vi "NonLinearPidTuningPanel.vi"() -> (3 "Output":string)   [LabVIEW 2014]
uses:
  <vilib>/silver_ctls/ArrayMatrixCluster/Real Matrix NI_Silver.ctl
panel:
  in  "Matrix Type":u16(ring) items=["Diagonal", "Normal"]
  in  "K anti wind up":T1=[[2.0, 0.0, 0.0, 0.0, 0.0, 0.0], [0.0, 1.0, 0.0, 0.0, 0.0, 0.0], [0.0, 0.0, 2.0, 0.0, 0.0, 0.0], [0.0, 0.0, 0.0, 0.0, 0.0, 0.0], [0.0, 0.0, 0.0, 0.0, 0.0, 0.0], [0.0, 0.0, 0.0, 0.0, 0.0, 1.0]]
  in  "Ki":T1=[[10.0, 0.0, 0.0, 0.0, 0.0, 0.0], [0.0, 10.0, 0.0, 0.0, 0.0, 0.0], [0.0, 0.0, 20.0, 0.0, 0.0, 0.0], [0.0, 0.0, 0.0, 0.0, 0.0, 0.0], [0.0, 0.0, 0.0, 0.0, 0.0, 0.0], [0.0, 0.0, 0.0, 0.0, 0.0, 5.0]]
  in  "Kd":T1=[[400.0, 0.0, 0.0, 0.0, 0.0, 0.0], [0.0, 400.0, 0.0, 0.0, 0.0, 0.0], [0.0, 0.0, 400.0, 0.0, 0.0, 0.0], [0.0, 0.0, 0.0, 0.0, 0.0, 0.0], [0.0, 0.0, 0.0, 0.0, 0.0, 0.0], [0.0, 0.0, 0.0, 0.0, 0.0, 200.0]]
  in  "Kp":T1=[[300.0, 0.0, 0.0, 0.0, 0.0, 0.0], [0.0, 300.0, 0.0, 0.0, 0.0, 0.0], [0.0, 0.0, 500.0, 0.0, 0.0, 0.0], [0.0, 0.0, 0.0, 0.0, 0.0, 0.0], [0.0, 0.0, 0.0, 0.0, 0.0, 0.0], [0.0, 0.0, 0.0, 0.0, 0.0, 200.0]]
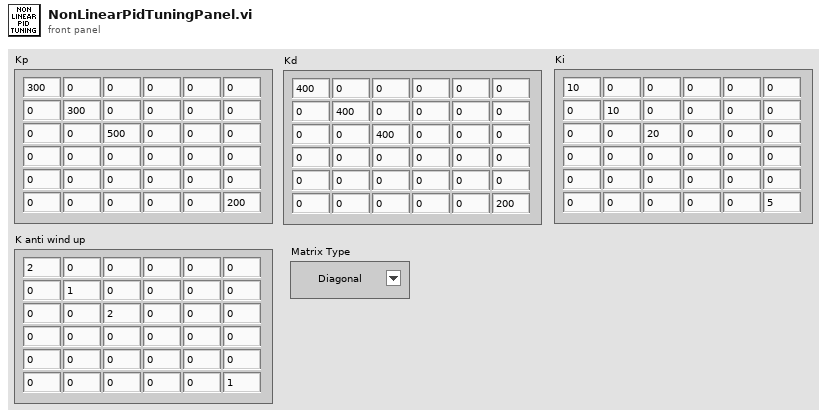
[diagram p1: front panel]
types:
  T1 = typedef "Real Matrix NI_Silver.ctl" = dbl[][]
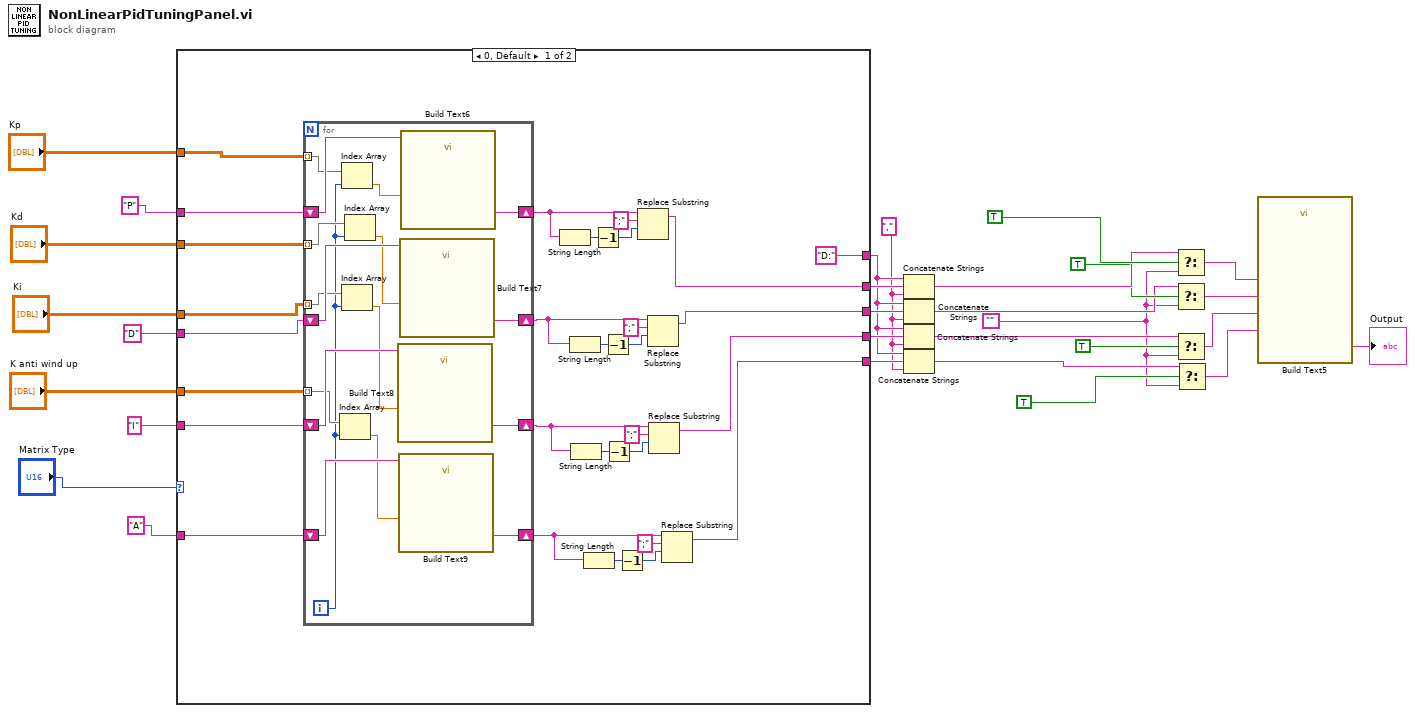
[diagram p0: block diagram]
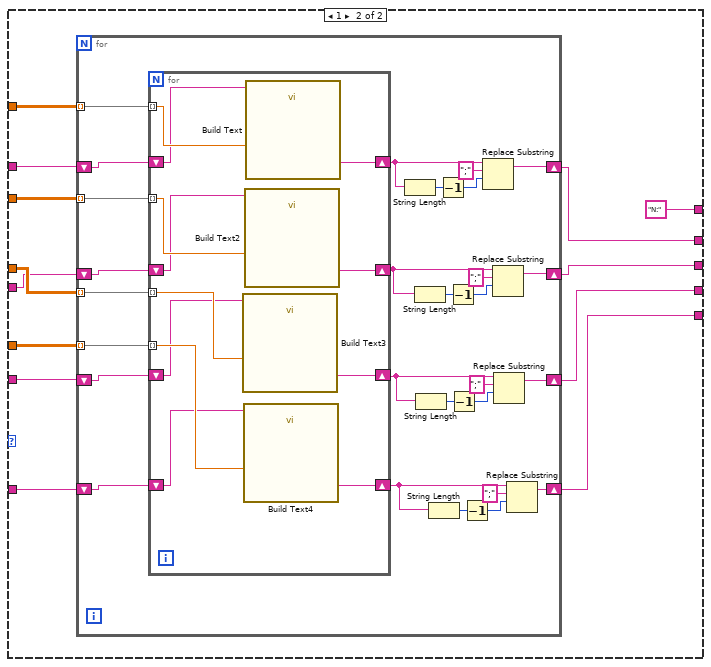
[diagram p2: hidden frame]
diagram:
  w2 = ","
  w1 = ""
  n1 = case shown="0, Default" "Matrix Type" {
    tunnel: "Kp" -> [w42 w88]
    tunnel: "Kd" -> [w41 w87]
    tunnel: "Ki" -> [w40 w86]
    tunnel: "K anti wind up" -> [w39 w85]
    tunnel: [w38 w84] -> w23
    tunnel: [w37 w83] -> w22
    tunnel: [w36 w82] -> w21
    tunnel: [w35 w81] -> w20
    tunnel: ["D:" "N:"] -> w19
    tunnel: "P" -> [w33 w79]
    tunnel: "D" -> [w32 w78]
    tunnel: "A" -> [w31 w76]
    tunnel: "I" -> [w30 w77]
    frame 0, Default {
      n2 = for {
        tunnel: w42 -> [w67] mode=indexing
        shift-right: [w75] -> w43
        shift-left: w31 -> [w74]
        shift-right: [w73] -> w44
        shift-left: w30 -> [w72]
        shift-right: [w71] -> w45
        shift-left: w32 -> [w70]
        shift-right: [w69] -> w58
        shift-left: w33 -> [w68]
        tunnel: w41 -> [w65] mode=indexing
        tunnel: w40 -> [w63] mode=indexing
        tunnel: w39 -> [w61] mode=indexing
        i -> [w60]
        n3 = Index Array(array=w61, index=w60) -> (element=w59:dbl)
        n4 = Index Array(array=w67, index=w60) -> (element=w66:dbl)
        n5 = Index Array(array=w63, index=w60) -> (element=w62:dbl)
        n6 = Index Array(array=w65, index=w60) -> (element=w64:dbl)
        n7 = call "Build Text8"("Beginning Text"=w72, "Elem"=w62) -> ("Result"=w73:string)  [unwired: 12 in, 1 out]
        n8 = call "Build Text9"("Beginning Text"=w74, "Elem"=w59) -> ("Result"=w75:string)  [unwired: 12 in, 1 out]
        n9 = call "Build Text7"("Beginning Text"=w70, "Elem"=w64) -> ("Result"=w71:string)  [unwired: 12 in, 1 out]
        n10 = call "Build Text6"("Beginning Text"=w68, "Elem"=w66) -> ("Result"=w69:string)  [unwired: 12 in, 1 out]
      }
      n11 = String Length(string=w58) -> (length=w56:i32)
      n12 = String Length(string=w45) -> (length=w53:i32)
      n13 = String Length(string=w44) -> (length=w50:i32)
      n14 = String Length(string=w43) -> (length=w47:i32)
      n15 = Decrement(x=w56) -> (x-1=w55:i32)
      n16 = Decrement(x=w53) -> (x-1=w52:i32)
      n17 = Decrement(x=w50) -> (x-1=w49:i32)
      n18 = Decrement(x=w47) -> (x-1=w46:i32)
      n19 = Replace Substring(3:w55, 4:";" ("substring (\"\")"), 5:w58) -> (1:w38:string)  [unwired: 1 in, 1 out]
      n20 = Replace Substring(3:w52, 4:";" ("substring (\"\")"), 5:w45) -> (1:w37:string)  [unwired: 1 in, 1 out]
      n21 = Replace Substring(3:w49, 4:";" ("substring (\"\")"), 5:w44) -> (1:w36:string)  [unwired: 1 in, 1 out]
      n22 = Replace Substring(3:w46, 4:";" ("substring (\"\")"), 5:w43) -> (1:w35:string)  [unwired: 1 in, 1 out]
    }
    frame 1 {
      n23 = for {
        tunnel: w88 -> [w116] mode=indexing
        tunnel: w87 -> [w115] mode=indexing
        tunnel: w86 -> [w114] mode=indexing
        tunnel: w85 -> [w113] mode=indexing
        shift-right: [w108] -> w84
        shift-left: w79 -> [w107]
        shift-right: [w96] -> w83
        shift-left: w78 -> [w95]
        shift-right: [w94] -> w82
        shift-left: w77 -> [w93]
        shift-right: [w92] -> w81
        shift-left: w76 -> [w91]
        n24 = for {
          tunnel: w116 -> [w128] mode=indexing
          tunnel: w115 -> [w127] mode=indexing
          tunnel: w114 -> [w126] mode=indexing
          tunnel: w113 -> [w125] mode=indexing
          shift-right: [w124] -> w89
          shift-left: w91 -> [w123]
          shift-right: [w122] -> w90
          shift-left: w93 -> [w121]
          shift-right: [w120] -> w97
          shift-left: w95 -> [w119]
          shift-right: [w118] -> w112
          shift-left: w107 -> [w117]
          n25 = call "Build Text3"("Beginning Text"=w121, "Elem"=w126) -> ("Result"=w122:string)  [unwired: 12 in, 1 out]
          n26 = call "Build Text4"("Beginning Text"=w123, "Elem"=w125) -> ("Result"=w124:string)  [unwired: 12 in, 1 out]
          n27 = call "Build Text2"("Beginning Text"=w119, "Elem"=w127) -> ("Result"=w120:string)  [unwired: 12 in, 1 out]
          n28 = call "Build Text"("Beginning Text"=w117, "Elem"=w128) -> ("Result"=w118:string)  [unwired: 12 in, 1 out]
        }
        n29 = String Length(string=w112) -> (length=w110:i32)
        n30 = String Length(string=w97) -> (length=w105:i32)
        n31 = String Length(string=w90) -> (length=w102:i32)
        n32 = String Length(string=w89) -> (length=w99:i32)
        n33 = Decrement(x=w110) -> (x-1=w109:i32)
        n34 = Decrement(x=w105) -> (x-1=w104:i32)
        n35 = Decrement(x=w102) -> (x-1=w101:i32)
        n36 = Decrement(x=w99) -> (x-1=w98:i32)
        n37 = Replace Substring(3:w109, 4:";" ("substring (\"\")"), 5:w112) -> (1:w108:string)  [unwired: 1 in, 1 out]
        n38 = Replace Substring(3:w104, 4:";" ("substring (\"\")"), 5:w97) -> (1:w96:string)  [unwired: 1 in, 1 out]
        n39 = Replace Substring(3:w101, 4:";" ("substring (\"\")"), 5:w90) -> (1:w94:string)  [unwired: 1 in, 1 out]
        n40 = Replace Substring(3:w98, 4:";" ("substring (\"\")"), 5:w89) -> (1:w92:string)  [unwired: 1 in, 1 out]
      }
    }
  }
  n41 = Concatenate Strings(w19, w23, w2) -> (w13:string)
  n42 = Concatenate Strings(w19, w22, w2) -> (w10:string)
  n43 = Concatenate Strings(w19, w21, w2) -> (w7:string)
  n44 = Concatenate Strings(w19, w20, w2) -> (w4:string)
  n45 = Select(t=w13, s=TRUE ("Update Kp"), f=w1) -> (s? t:f=w12:string)
  n46 = Select(t=w10, s=TRUE ("Update Kd"), f=w1) -> (s? t:f=w9:string)
  n47 = Select(t=w7, s=TRUE ("Update Ki"), f=w1) -> (s? t:f=w6:string)
  n48 = Select(t=w4, s=TRUE ("Update Ka"), f=w1) -> (s? t:f=w3:string)
  n49 = call "Build Text5"("Kanti"=w3, "Kp"=w12, "Kd"=w9, "Ki"=w6) -> ("Result"=→"Output":string)  [unwired: 10 in, 1 out]
